vi "KepcoDCPwr Configure OVP.vi"(0 "VISA Session":refnum<visa-resource-name>, 5 "Model In":string, 7 "channel name (\"\")":string="\"\"", 9 "limit (0.0 volts)":dbl format="%^.2e", 11 "error in (no error)":errorcluster {"code" format="%.0x"}, 12 "enabled (False)":bool) -> (4 "VISA Session Out":refnum<visa-resource-name>, 6 "Model Out":string, 8 "channel name out (\"\")":string="\"\"" caption="channel name Out (\"\")", 15 "error out":errorcluster {"code" format="%.0x"})   [LabVIEW 2010]
doc: "This VI configures the power supply's over-voltage protection.\n\nWhen the enabled parameter is FALSE, the driver sets the unit to its max over voltage protection limit."
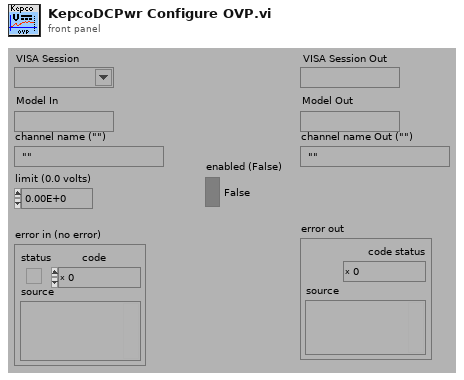
[diagram p1: front panel]
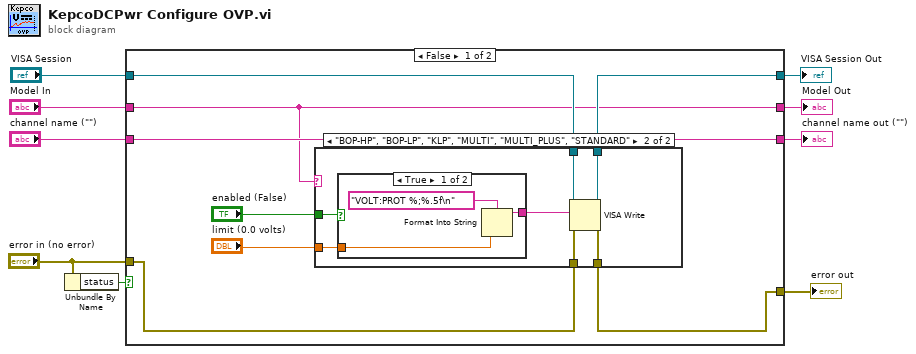
[diagram p0: block diagram]
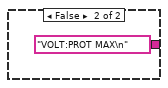
[diagram p3: hidden frame]
diagram:
  n1 = Unbundle By Name("error in (no error)") -> ("status"=w5:bool)
  n2 = case shown="False" w5 {
    tunnel: [w14 w33] -> w9
    tunnel: [w15 w34] -> w7
    tunnel: "VISA Session" -> [w16 w34]
    tunnel: "error in (no error)" -> [w13 w33]
    tunnel: "Model In" -> [w12 w32]
    tunnel: "channel name (\"\")" -> [w17 w31]
    tunnel: [w12 w32] -> w2
    tunnel: [w17 w31] -> w1
    frame False {
      n3 = case shown="\"BOP-HP\", \"BOP-LP\", \"KLP\", \"MULTI\", \"MULTI_PLUS\", \"STANDARD\"" w12 {
        tunnel: w13 -> [w19 w26]
        tunnel: [w19 w25] -> w14
        tunnel: w16 -> [w18 w24]
        tunnel: [w18 w23] -> w15
        tunnel: "limit (0.0 volts)" -> [_ w22]
        tunnel: "enabled (False)" -> [_ w20]
        frame "", Default {
        }
        frame "BOP-HP", "BOP-LP", "KLP", "MULTI", "MULTI_PLUS", "STANDARD" {
          n4 = case shown="True" w20 {
            tunnel: w22 -> [w27 _]
            tunnel: [w28 "VOLT:PROT MAX\n"] -> w21
            frame True {
              n5 = Format Into String(format string="VOLT:PROT %;%.5f\n", w27) -> (resulting string=w28:string)  [unwired: 2 in, 1 out]
            }
            frame False {
            }
          }
          n6 = VISA Write(VISA resource name=w24, write buffer=w21, error in (no error)=w26) -> (VISA resource name out=w23:refnum<visa-resource-name>, error out=w25:errorcluster)  [unwired: 1 out]
        }
      }
    }
    frame True {
    }
  }
  "error out" <- w9
  "VISA Session Out" <- w7
  "Model Out" <- w2
  "channel name out (\"\")" <- w1
